vi "image-viewer.vi"(10 "tif pointer":i64 format="%x") -> ()   [LabVIEW 2013]
uses:
  <vilib>/picture/picture.llb/imagedata.ctl
  imagereconstruction/x64/Debug/labviewdll.dll
panel:
  out "image data":T1
  out "error":i32
  in  "img num":i32
  in  "stop":bool
  out "new picture":picture
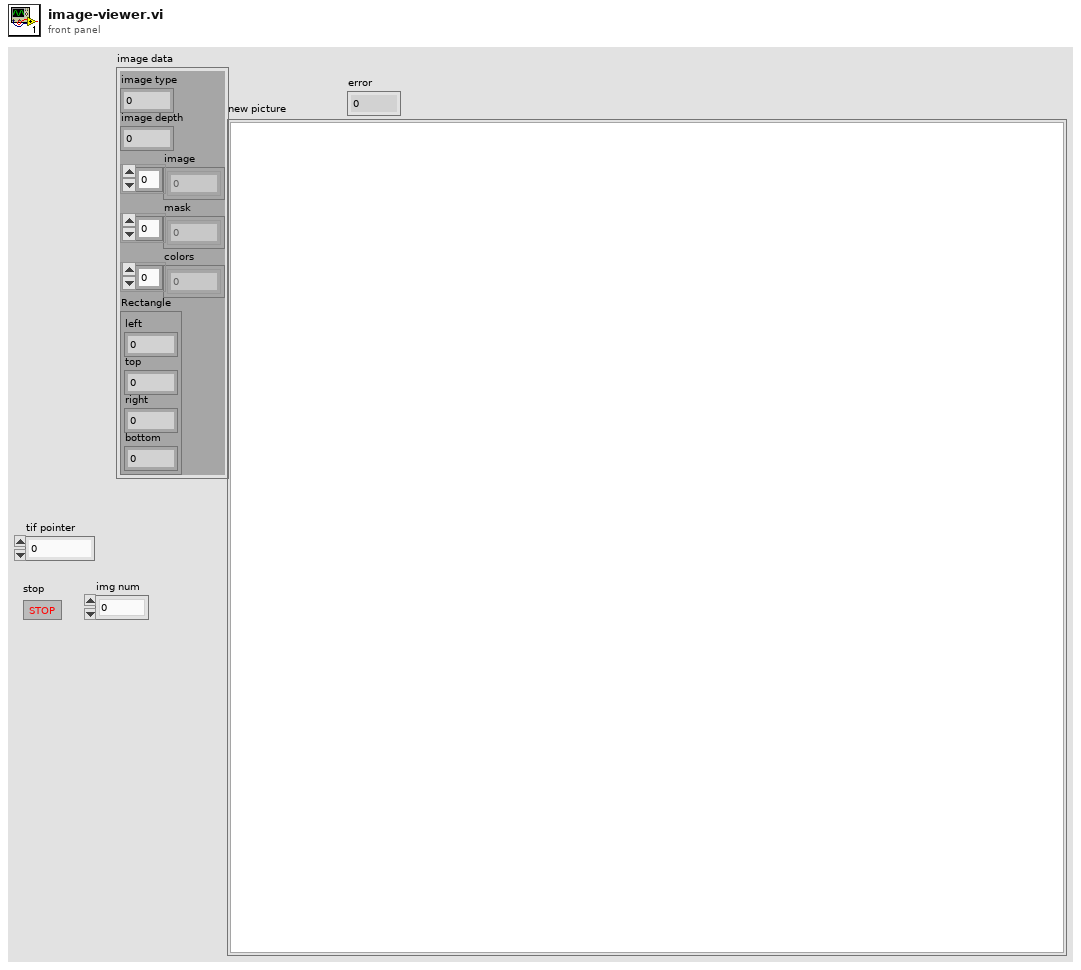
[diagram p1: front panel]
types:
  T1 = typedef "imagedata.ctl" = cluster{"image type":i32, "image depth":i32, "image":u8[], "mask":u8[], "colors":u32[], "Rectangle":cluster{"left":i16, "top":i16, "right":i16, "bottom":i16}}
  T2 = typedef "tags_cluster.ctl" = cluster{"compression":i32, "image width":i32, "image length":i32, "host computer":string, "software":string, "bitness":i32, "number of pages":i32, "samples per pixel":i32, "scanline size":i32, "strip size":i32, "lines per strip":i32}
  T3 = cluster{"left":i16, "top":i16, "right":i16, "bottom":i16}
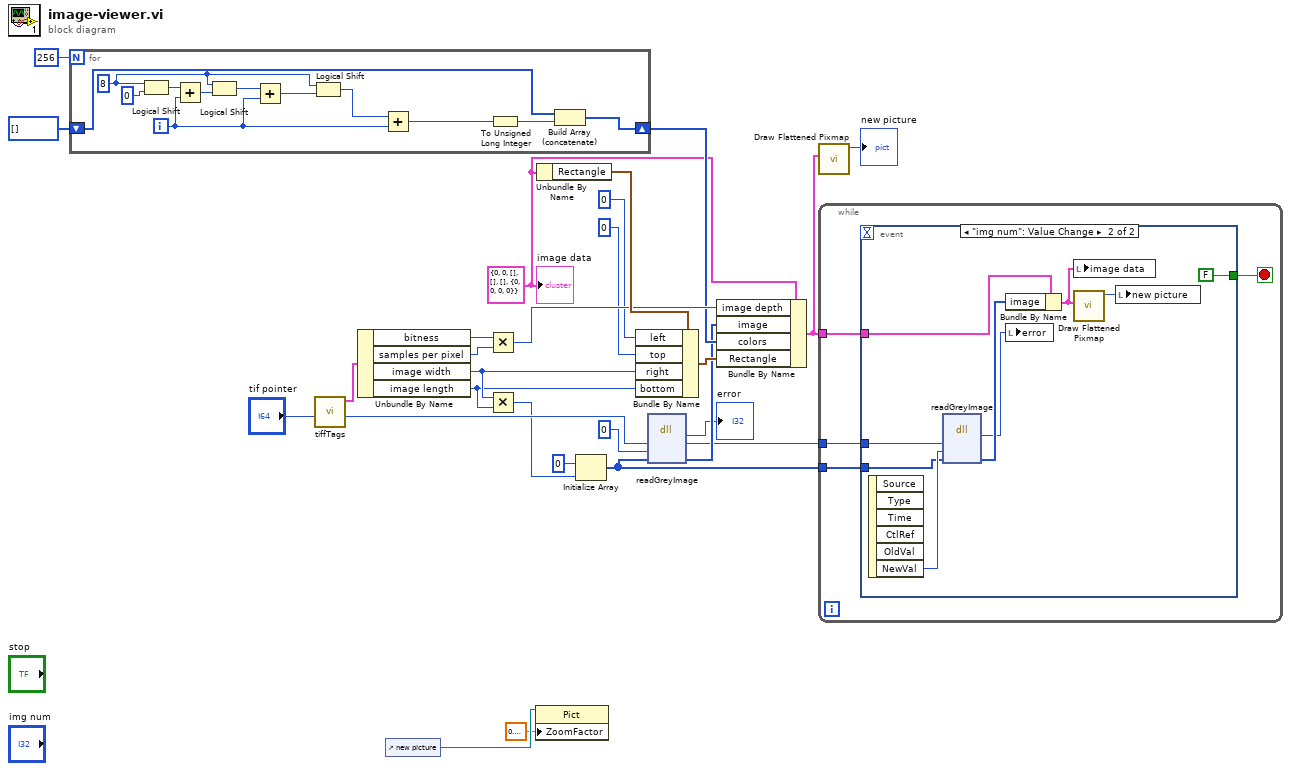
[diagram p0: block diagram]
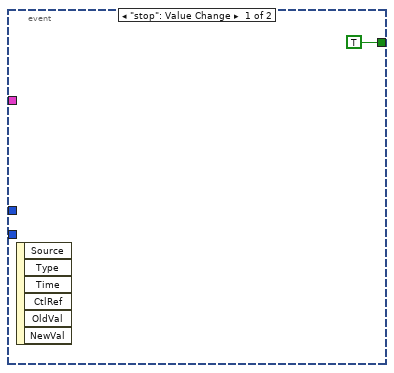
[diagram p2: hidden frame]
diagram:
  w3 = T1 {"image type"=0, "image depth"=0, "image"=[], "mask"=[], "colors"=[], "Rectangle"={"left"=0, "top"=0, "right"=0, "bottom"=0}} ("image data")
  n1 = for {
    N: 256 -> [_]
    shift-right: [w38] -> w18
    shift-left: u32[] [] -> [w39]
    i -> [w29]
    w32 = i16 8 ("y")
    n2 = Logical Shift(y=w32, x=u32 0) -> (x << y=w35:u32)
    n3 = Add(x=w35, y=w29) -> (x+y=w36:u32)
    n4 = Logical Shift(y=w32, x=w36) -> (x << y=w34:u32)
    n5 = Add(x=w34, y=w29) -> (x+y=w33:u32)
    n6 = Logical Shift(y=w32, x=w33) -> (x << y=w31:u32)
    n7 = Add(x=w31, y=w29) -> (x+y=w30:u32)
    n8 = To Unsigned Long Integer(number=w30) -> (unsigned 32bit integer=w37:u32)
    n9 = Build Array (concatenate)(w39, w37) -> (w38:u32[])
  }
  n10 = call "tiffTags.vi"("tif pointer"="tif pointer") -> ("tiff pointer"=w15:i64, "Image Properties"=w16:T2)  [unwired: 8 in, 1 out]
  n11 = Unbundle By Name(w16) -> ("bitness"=w23:i32, "samples per pixel"=w24:i32, "image width"=w13:i32, "image length"=w12:i32)
  n12 = control-ref of="new picture"() -> (w2:refnum<vi>)
  n13 = Multiply(x=w23, y=w24) -> (x*y=w22:i32)
  n14 = Multiply(x=w13, y=w12) -> (x*y=w14:i32)
  n15 = property class="Pict"(reference=w2, "ZoomFactor"=sgl 0.4 ("Zoom Factor")) -> ()  [unwired: 1 in, 2 out]
  n16 = Unbundle By Name(w3) -> ("Rectangle"=w26:T3)
  n17 = Initialize Array(u8 0 ("element"), w14) -> (w6:u8[])
  n18 = Bundle By Name(cluster=w26, "left"=i16 0, "top"=i16 0, "right"=w13, "bottom"=w12) -> (w25:T3)
  n19 = dll-call lib="D:/work/uni/FYP/reconrepo/imagereconstruction/x64/Debug/labviewdll.dll" fn="readGreyImage"("tiff"=w15, "directory"=0, "buffer"=w6) -> ("return type"=→"error":i32, "tiff"=w7:i64, "buffer"=w8:u8[])  [unwired: 4 in, 2 out]
  n20 = Bundle By Name(cluster=w3, "image depth"=w22, "image"=w8, "colors"=w18, "Rectangle"=w25) -> (w5:T1)
  n21 = call <vilib>:"Draw Flattened Pixmap.vi"("image data"=w5) -> ("new picture"=→"new picture":picture)  [unwired: 8 in]
  n22 = while {
    tunnel: w7 -> [w43]
    tunnel: w6 -> [w42]
    tunnel: w5 -> [w41]
    stop <- w40 stop-if-true
    n23 = event shown="[1] \"img num\": Value Change" {
      selector: _ -> [_ _]
      dyn-events: _ -> [_ _]
      timeout: _ -> [_ _]
      tunnel: w43 -> [_ w52]
      tunnel: [TRUE FALSE] -> w40
      tunnel: w42 -> [_ w50]
      tunnel: w41 -> [_ w48]
      event "stop": Value Change {
        n24 = event-data() -> ()  [unwired: 1 in, 6 out]
      }
      event "img num": Value Change {
        n25 = event-data() -> ("NewVal"=w51:i32)  [unwired: 1 in, 5 out]
        n26 = dll-call lib="D:/work/uni/FYP/reconrepo/imagereconstruction/x64/Debug/labviewdll.dll" fn="readGreyImage"("tiff"=w52, "directory"=w51, "buffer"=w50) -> ("return type"=w46:i32, "buffer"=w49:u8[])  [unwired: 5 in, 2 out]
        n27 = Bundle By Name(cluster=w48, "image"=w49) -> (w45:T1)
        n28 = local write "error"(w46) -> ()
        n29 = local write "image data"(w45) -> ()
        n30 = call <vilib>:"Draw Flattened Pixmap.vi"("image data"=w45) -> ("new picture"=w47:picture)  [unwired: 8 in]
        n31 = local write "new picture"(w47) -> ()
      }
    }
  }
  "image data" <- w3
